vi "RandomIndex.vi"(10 "Nbre de valeur":i32=5, 11 "Taille du tab":i32=7) -> (2 "RandomComplementaryIndex":i32[](array[numeric]), 3 "RandomIndex":i32[](array[numeric]))   [LabVIEW 2020]
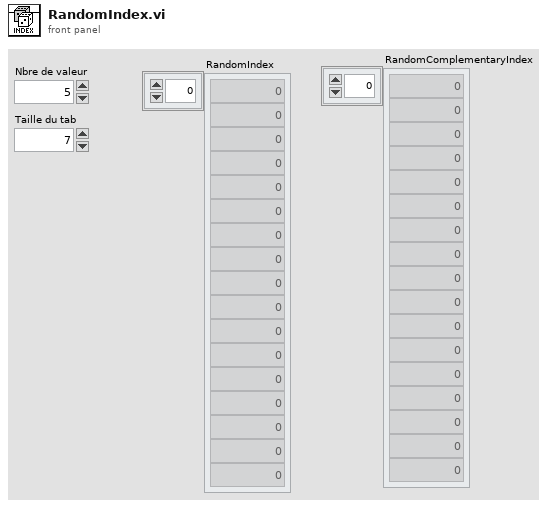
[diagram p1: front panel]
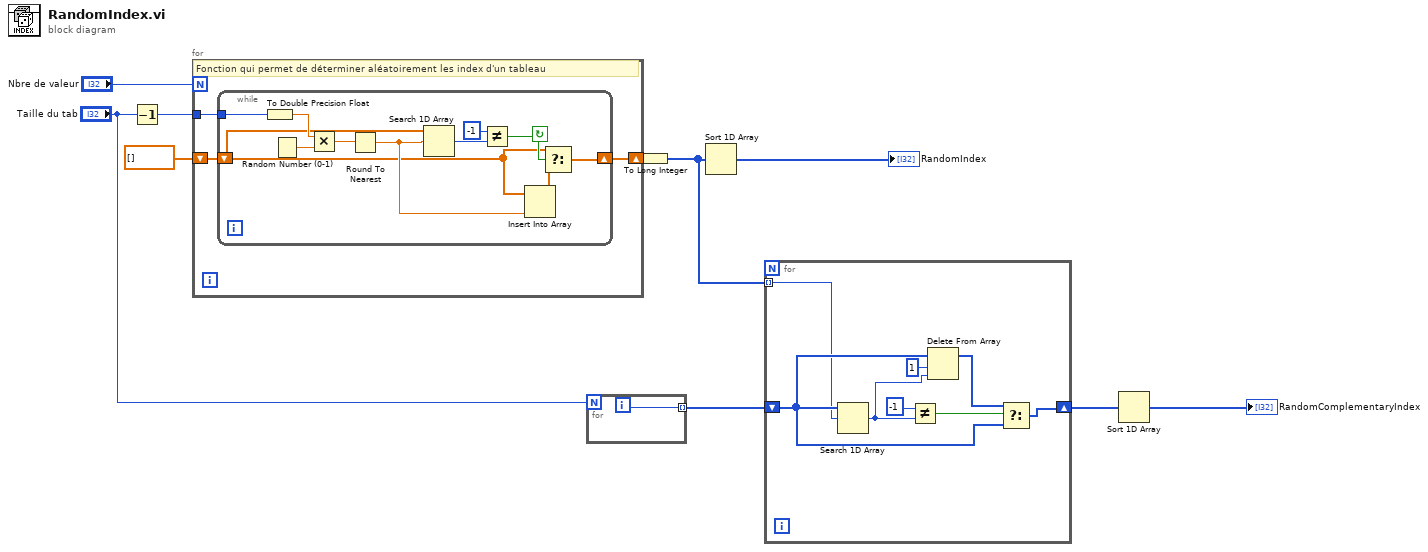
[diagram p0: block diagram]
diagram:
  n1 = Decrement(x="Taille du tab") -> (x-1=w1:i32)
  n2 = for {
    N: "Nbre de valeur" -> [_]
    tunnel: w1 -> [w13]
    shift-right: [w11] -> w7
    shift-left: dbl[] [] ("Array") -> [w12]
    # "Fonction qui permet de déterminer aléatoirement les index d'un tableau"
    n3 = while {
      tunnel: w13 -> [w24]
      shift-right: [w16] -> w11
      shift-left: w12 -> [w14]
      stop <- w17 continue-if-true
      n4 = To Double Precision Float(number=w24) -> (double precision float=w22:dbl)
      n5 = Random Number (0-1)() -> (number: 0 to 1=w23:dbl)
      n6 = Multiply(x=w22, y=w23) -> (x*y=w21:dbl)
      n7 = Round To Nearest(number=w21) -> (nearest integer value=w18:dbl)
      n8 = Search 1D Array(1D array=w14, element=w18) -> (index of element=w20:i32)  [unwired: 1 in]
      n9 = Not Equal?(x=-1, y=w20) -> (x != y?=w17:bool)
      n10 = Insert Into Array(array=w14, new element=w18) -> (w15:dbl[])  [unwired: 1 in]
      n11 = Select(t=w14, s=w17, f=w15) -> (s? t:f=w16:dbl[])
    }
  }
  n12 = for {
    N: "Taille du tab" -> [_]
    tunnel: [w25] -> w6 mode=indexing
    i -> [w25]
  }
  n13 = To Long Integer(number=w7) -> (32bit integer=w5:i32[])
  n14 = Sort 1D Array(array=w5) -> (sorted array=→"RandomIndex":i32[])
  n15 = for {
    tunnel: w5 -> [w26] mode=indexing
    shift-right: [w32] -> w4
    shift-left: w6 -> [w30]
    n16 = Search 1D Array(1D array=w30, element=w26) -> (index of element=w28:i32)  [unwired: 1 in]
    n17 = Not Equal?(x=-1, y=w28) -> (x != y?=w33:bool)
    n18 = Delete From Array(array=w30, length=1, index=w28) -> (array with subset deleted=w27:i32[])  [unwired: 1 out]
    n19 = Select(t=w27, s=w33, f=w30) -> (s? t:f=w32:i32[])
  }
  n20 = Sort 1D Array(array=w4) -> (sorted array=→"RandomComplementaryIndex":i32[])
